vi "add_node.vi"(6 "ControlPaths":path, 7 "Node Type":T1, 8 "error in (no error)":errorcluster, 9 "Number of Parameters":i32=1, 10 "BD Position":cluster{"Left":i32, "Top":i32}={"Left"=75, "Top"=60}, 11 "VI Ref In":refnum<vi>) -> (0 "error out":errorcluster, 2 "Node Refnum":refnum<vi>, 3 "VI Ref Out":refnum<vi>)   [LabVIEW 2018]
uses:
  TypeDefinitions/node_types.ctl
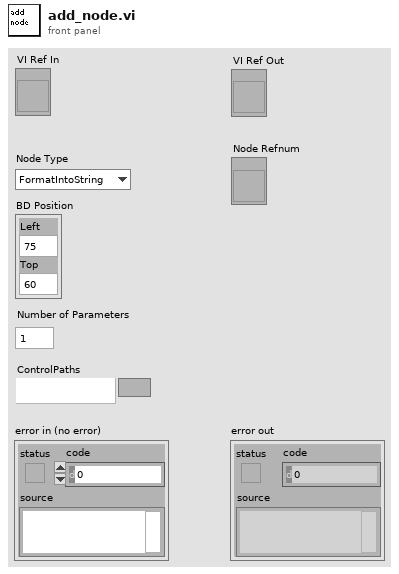
[diagram p1: front panel]
types:
  T1 = typedef "node_types.ctl" = enum16{"FormatIntoString", "PickLine", "AppendTrueFalse", "VISAWrite", "SubVI", "ConcatenateStrings", "VISARead", "ProperyNode", "ScanFromString", "SpreadSheetStringToArray"}
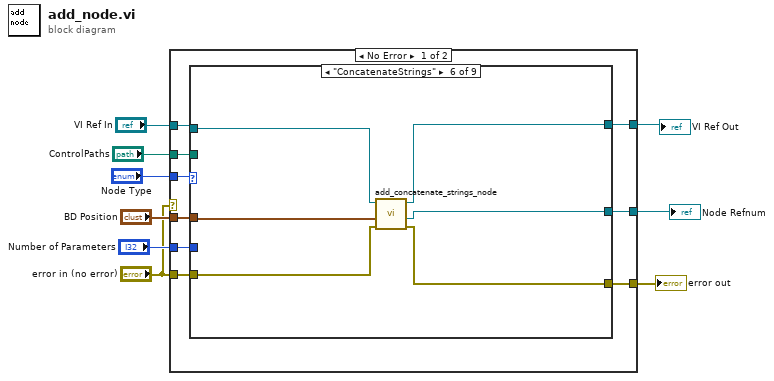
[diagram p0: block diagram]
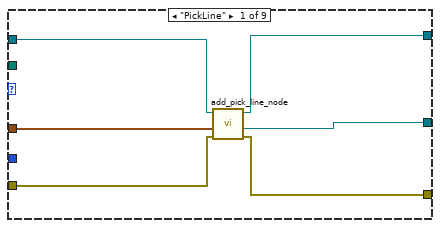
[diagram p2: hidden frame]
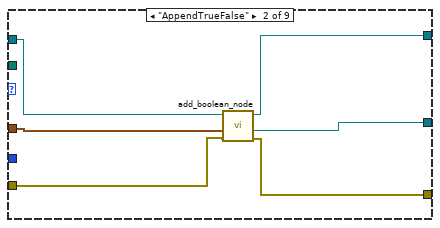
[diagram p3: hidden frame]
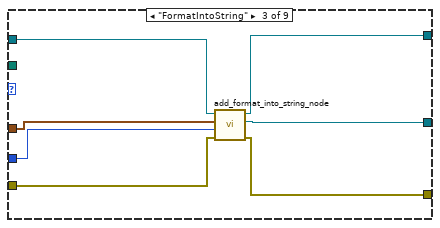
[diagram p4: hidden frame]
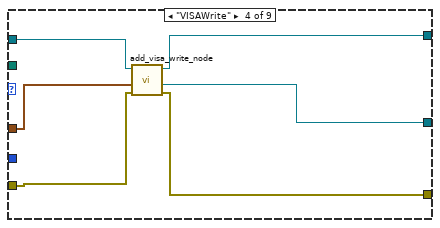
[diagram p5: hidden frame]
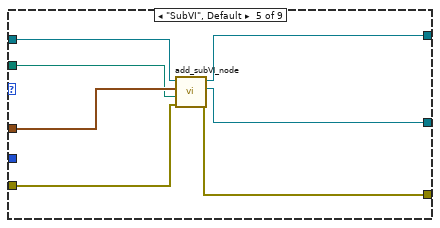
[diagram p6: hidden frame]
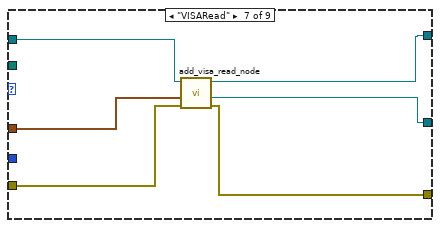
[diagram p7: hidden frame]
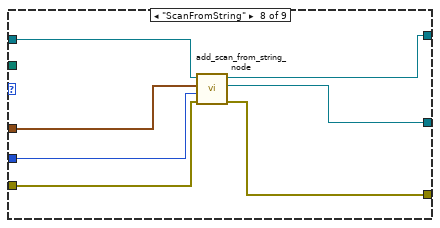
[diagram p8: hidden frame]
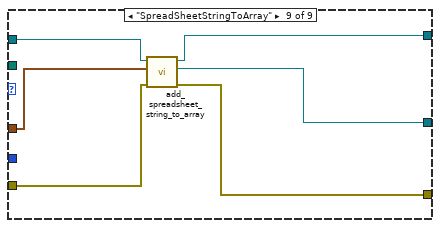
[diagram p9: hidden frame]
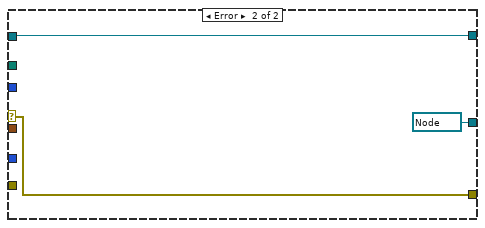
[diagram p10: hidden frame]
diagram:
  n1 = case shown="No Error" "error in (no error)" {
    selector: "error in (no error)" -> [_ w78]
    tunnel: "Node Type" -> [w18 _]
    tunnel: [w17 w78] -> w8
    tunnel: "error in (no error)" -> [w16 _]
    tunnel: "VI Ref In" -> [w15 w77]
    tunnel: [w14 w77] -> w6
    tunnel: [w13 refnum<vi> refnum ("Node Refnum")] -> w5
    tunnel: "BD Position" -> [w12 _]
    tunnel: "Number of Parameters" -> [w11 _]
    tunnel: "ControlPaths" -> [w10 _]
    frame No Error {
      n2 = case shown="\"ConcatenateStrings\"" w18 {
        tunnel: w15 -> [w24 w30 w37 w43 w50 w56 w58 w69 w75]
        tunnel: [w23 w29 w36 w39 w49 w53 w57 w67 w73] -> w14
        tunnel: [w22 w27 w32 w40 w47 w51 w60 w65 w70] -> w17
        tunnel: w16 -> [w21 w26 w33 w41 w46 w54 w61 w64 w71]
        tunnel: [w20 w28 w35 w38 w48 w52 w59 w66 w72] -> w13
        tunnel: w12 -> [w19 w25 w34 w42 w45 w55 w62 w68 w74]
        tunnel: w11 -> [_ _ w31 _ _ _ _ w63 _]
        tunnel: w10 -> [_ _ _ _ w44 _ _ _ _]
        frame "PickLine" {
          n3 = call "add_pick_line_node.vi"("error in (no error)"=w21, "BD Position"=w19, "VI Ref In"=w24) -> ("error out"=w22:errorcluster, "Node Refnum"=w20:refnum<vi>, "VI Ref Out"=w23:refnum<vi>)  [unwired: 6 out]
        }
        frame "AppendTrueFalse" {
          n4 = call "add_boolean_node.vi"("error in (no error)"=w26, "BD Position"=w25, "VI Ref In"=w30) -> ("error out"=w27:errorcluster, "Node Refnum"=w28:refnum<vi>, "VI Ref Out"=w29:refnum<vi>)  [unwired: 6 out]
        }
        frame "FormatIntoString" {
          n5 = call "add_format_into_string_node.vi"("error in (no error)"=w33, "Number of Parameters"=w31, "BD Position"=w34, "VI Ref In"=w37) -> ("error out"=w32:errorcluster, "Node Refnum"=w35:refnum<vi>, "VI Ref Out"=w36:refnum<vi>)  [unwired: 5 out]
        }
        frame "VISAWrite" {
          n6 = call "add_visa_write_node.vi"("error in (no error)"=w41, "BD Position"=w42, "VI Ref In"=w43) -> ("error out"=w40:errorcluster, "Node Refnum"=w38:refnum<vi>, "VI Ref Out"=w39:refnum<vi>)  [unwired: 6 out]
        }
        frame "SubVI", Default {
          n7 = call "add_subVI_node.vi"("error in"=w46, "ControlPaths"=w44, "ControlPosition"=w45, "VI Ref In"=w50) -> ("error out"=w47:errorcluster, "SubVI Refnum Out"=w48:refnum<vi>, "VI Ref Out"=w49:refnum<vi>)  [unwired: 5 out]
        }
        frame "ConcatenateStrings" {
          n8 = call "add_concatenate_strings_node.vi"("error in (no error)"=w54, "BD Position"=w55, "VI Ref In"=w56) -> ("error out"=w51:errorcluster, "Node Refnum"=w52:refnum<vi>, "VI Ref Out"=w53:refnum<vi>)  [unwired: 6 out]
        }
        frame "VISARead" {
          n9 = call "add_visa_read_node.vi"("error in (no error)"=w61, "BD Position"=w62, "VI Ref In"=w58) -> ("error out"=w60:errorcluster, "Node Refnum"=w59:refnum<vi>, "VI Ref Out"=w57:refnum<vi>)  [unwired: 6 out]
        }
        frame "ScanFromString" {
          n10 = call "add_scan_from_string_node.vi"("error in (no error)"=w64, "Number of Parameters"=w63, "BD Position"=w68, "VI Ref In"=w69) -> ("error out"=w65:errorcluster, "Node Refnum"=w66:refnum<vi>, "VI Ref Out"=w67:refnum<vi>)  [unwired: 5 out]
        }
        frame "SpreadSheetStringToArray" {
          n11 = call "add_spreadsheet_string_to_array.vi"("error in (no error)"=w71, "BD Position"=w74, "VI Ref In"=w75) -> ("error out"=w70:errorcluster, "Node Refnum"=w72:refnum<vi>, "VI Ref Out"=w73:refnum<vi>)  [unwired: 6 out]
        }
      }
    }
    frame Error {
    }
  }
  "error out" <- w8
  "VI Ref Out" <- w6
  "Node Refnum" <- w5
